vi "DMD_sample.vi"() -> ()   [LabVIEW 2017]
panel:
  out "error out":errorcluster
  out "string":string
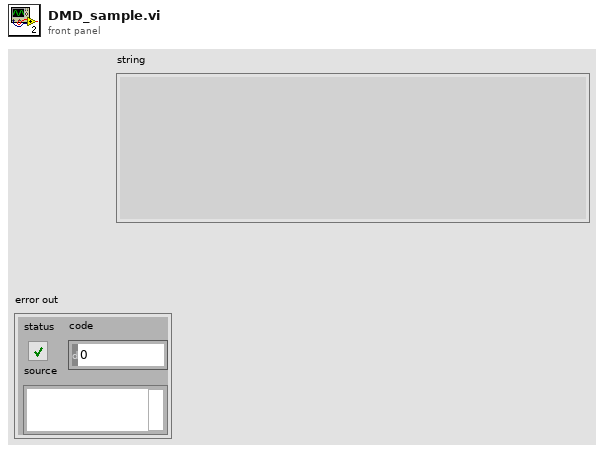
[diagram p1: front panel]
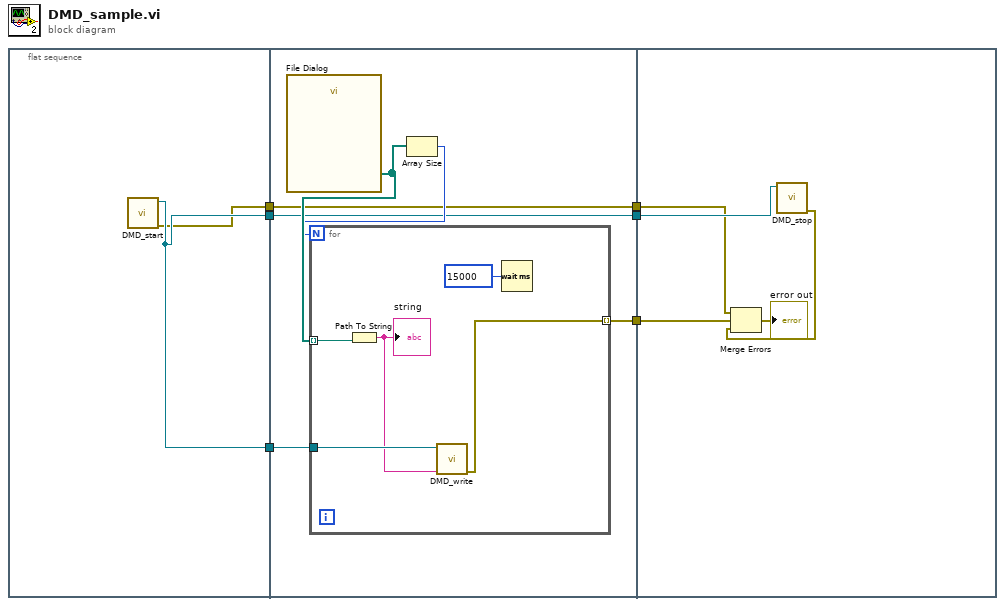
[diagram p0: block diagram]
diagram:
  n1 = flat-sequence {
    tunnel: [w8] -> w6
    tunnel: [w8] -> w4
    tunnel: [w7] -> w2
    tunnel: w6 -> [w12]
    tunnel: [w11] -> w5
    tunnel: w4 -> [w11]
    tunnel: [w10] -> w3
    tunnel: w2 -> [w10]
    tunnel: [w9] -> w1
    tunnel: w5 -> [w24]
    tunnel: w3 -> [w23]
    tunnel: w1 -> [w22]
    frame #0 {
      n2 = call "DMD_start.vi"() -> ("error out"=w7:errorcluster, "reference out"=w8:refnum<k24>)  [unwired: 10 in]
    }
    frame #1 {
      n3 = call "File Dialog"() -> ("selected paths"=w14:path[])  [unwired: 12 in, 3 out]
      n4 = Array Size(array=w14) -> (size(s)=w13:i32)
      n5 = for {
        N: w13 -> [_]
        tunnel: w14 -> [w19] mode=indexing
        tunnel: w12 -> [w18]
        tunnel: [w16] -> w9 mode=indexing
        n6 = Path To String(path=w19) -> (string=w17:string)
        "string" <- w17
        n7 = call "DMD_write.vi"("String"=w17, "reference out"=w18) -> ("error out"=w16:errorcluster)  [unwired: 9 in]
        n8 = Wait (ms)(milliseconds to wait=u32 15000) -> ()  [unwired: 1 out]
      }
    }
    frame #2 {
      n9 = call "DMD_stop.vi"("reference out"=w24) -> ("error out"=w21:errorcluster)  [unwired: 10 in]
      n10 = Merge Errors(w23, w22, w21) -> (→"error out":errorcluster)
    }
  }
